vi "ReadIEEE BlockUI1.vi"(7 "error in (no error)":errorcluster {"code" format="%.0x"}, 8 "ValBufferSize":i32=2048, 10 "instrument handle":refnum<k15>) -> (0 "error out":errorcluster {"code" format="%.0x"}, 1 "ValActualSize":i32, 3 "instrument handle out":refnum<k15>, 4 "Val":u8[](array[numeric]))   [LabVIEW 2014, in "Agilent NA.lvlib"]
doc: "Read definite-length IEEE binary block the I/O stream"
uses:
  Agilent NA.lvlib
  AgNA.dll
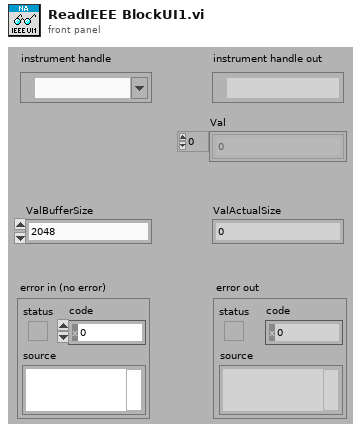
[diagram p1: front panel]
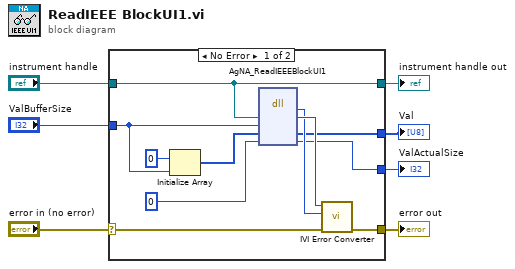
[diagram p0: block diagram]
diagram:
  n1 = case shown="No Error" "error in (no error)" {
    selector: "error in (no error)" -> [w16 w20]
    tunnel: [w15 w20] -> w7
    tunnel: "ValBufferSize" -> [w9 _]
    tunnel: [w13 _] -> w1
    tunnel: [w11 _] -> w4
    tunnel: [w10 w19] -> w3
    tunnel: "instrument handle" -> [w10 w19]
    frame No Error {
      n2 = Initialize Array(u8 0 ("element"), w9) -> (w8:u8[])
      n3 = dll-call lib="AgNA**.dll" fn="AgNA_ReadIEEEBlockUI1"("Vi"=w10, "ValBufferSize"=w9, "Val"=w8, "ValActualSize"=0) -> ("return type"=w17:i32, "Vi"=w18:u32, "Val"=w13:u8[], "ValActualSize"=w11:i32)  [unwired: 4 in, 2 out]
      n4 = call "IVI Error Converter.vi"("error in (no error)"=w16, "IVI error code (0)"=w17, "instrument handle"=w18) -> ("error out"=w15:errorcluster)  [unwired: 7 in, 1 out]
    }
    frame Error {
    }
  }
  "error out" <- w7
  "instrument handle out" <- w3
  "ValActualSize" <- w4
  "Val" <- w1
